vi "MGCC_StaEst_complex2magnitude.vi"(10 "st_MGCC_StaEst_Input":T1) -> (2 "output cluster":T1)   [LabVIEW 2016]
doc: "-----------------------------------------------------------------------------------------------------------------------\nCopyright <2019> <The University of Tennessee at Knoxville and the University of Tennessee Research Foundation>\nThis software is released under BSD-3 \nhttps://opensource.org/licenses/BSD-3-Clause \nAdditional license options available at https://utrf.tennessee.edu/industry/sample-agreements/\n-----------------------------------------------------------------------------------------------------------------------"
uses:
  Model Management/Global_MdlMgmt.vi
  Communication/Global communication.vi
  <vilib>/imath/engines/lvmath2/RunTimeEngine/IndexRead/NIMS M($,S).vi
  <instcachedir>/0/NIMS M($,S)_3E5749BBB62E49528D4765A77F1F6D98.lvgen/NIMS M($,S)_3E5749BBB62E49528D4765A77F1F6D98_000.vi
  <vilib>/imath/engines/lvmath2/RunTimeEngine/BuiltInFunctions/length/NIMS_length(GV).vi
  <instcachedir>/0/NIMS_length(GV)_08A3D13377FD4E4B96F5795FBF3698FA.lvgen/NIMS_length(GV)_08A3D13377FD4E4B96F5795FBF3698FA_000.vi
  <vilib>/imathl/engines/lvmath/Functions/Error Handling/Create Error.vi
  <vilib>/imath/engines/lvmath2/RunTimeEngine/RangeToken/NIMS_Range_R3 - Integer.vi
  <instcachedir>/0/NIMS_Range_R3 - Integer_A435E2FF893B4C718FD5055FE39FE2F6.lvgen/NIMS_Range_R3 - Integer_A435E2FF893B4C718FD5055FE39FE2F6_000.vi
  <vilib>/imath/engines/lvmath2/RunTimeEngine/CommandStatement/MC_CommandStatement_break.vi
  <vilib>/imath/engines/lvmath2/RunTimeEngine/IndexRead/NIMS M(S,S).vi
  <instcachedir>/0/NIMS M(S,S)_AC51E74150A542F7991B9634C66F3096.lvgen/NIMS M(S,S)_AC51E74150A542F7991B9634C66F3096_000.vi
  <vilib>/imath/engines/lvmath2/RunTimeSupport/NIMS_Error if Not Equal.vi
  <instcachedir>/0/NIMS_Error if Not Equal_43252A79AD05436189442EC0C5E5AB8A.lvgen/NIMS_Error if Not Equal_43252A79AD05436189442EC0C5E5AB8A_000.vi
  <vilib>/imath/engines/lvmath2/RunTimeEngine/IndexRead/NIMS V(S).vi
  <instcachedir>/0/NIMS V(S)_0488751826AF41519A22953C041130DC.lvgen/NIMS V(S)_0488751826AF41519A22953C041130DC_000.vi
  <vilib>/imath/engines/lvmath2/RunTimeEngine/IndexReplace/NIMS M(S,S)=S.vi
  <instcachedir>/0/NIMS M(S,S)=S_98E40400474E4398B113AE20298B4F82.lvgen/NIMS M(S,S)=S_98E40400474E4398B113AE20298B4F82_000.vi
  <vilib>/imath/engines/lvmath2/RunTimeEngine/ErrorHandling/NIMS_Create Error From Enums.vi
  <vilib>/imath/engines/lvmath2/RunTimeEngine/NodeEndStatement/NIMS_NodeEndStatement_Output.vi
  <instcachedir>/0/NIMS_NodeEndStatement_Output_53EC0D466D134D7ABD903AC30B43404B.lvgen/NIMS_NodeEndStatement_Output_53EC0D466D134D7ABD903AC30B43404B_002.vi
  <vilib>/imath/engines/lvmath2/RunTimeEngine/ErrorHandling/NIMS_Finalize Error.vi
  <vilib>/Utility/error.llb/Error Cluster From Error Code.vi
  <vilib>/ErrorRing/Error Ring.xnode
panel:
  out "error out":errorcluster
  out "appended array":dbl[][](array[numeric])
  out "V_node":cdb[][](array[numeric])
  out "r * e^(i*theta)":cdb[][](array[numeric])
  out "output array":dbl[][](array[numeric])
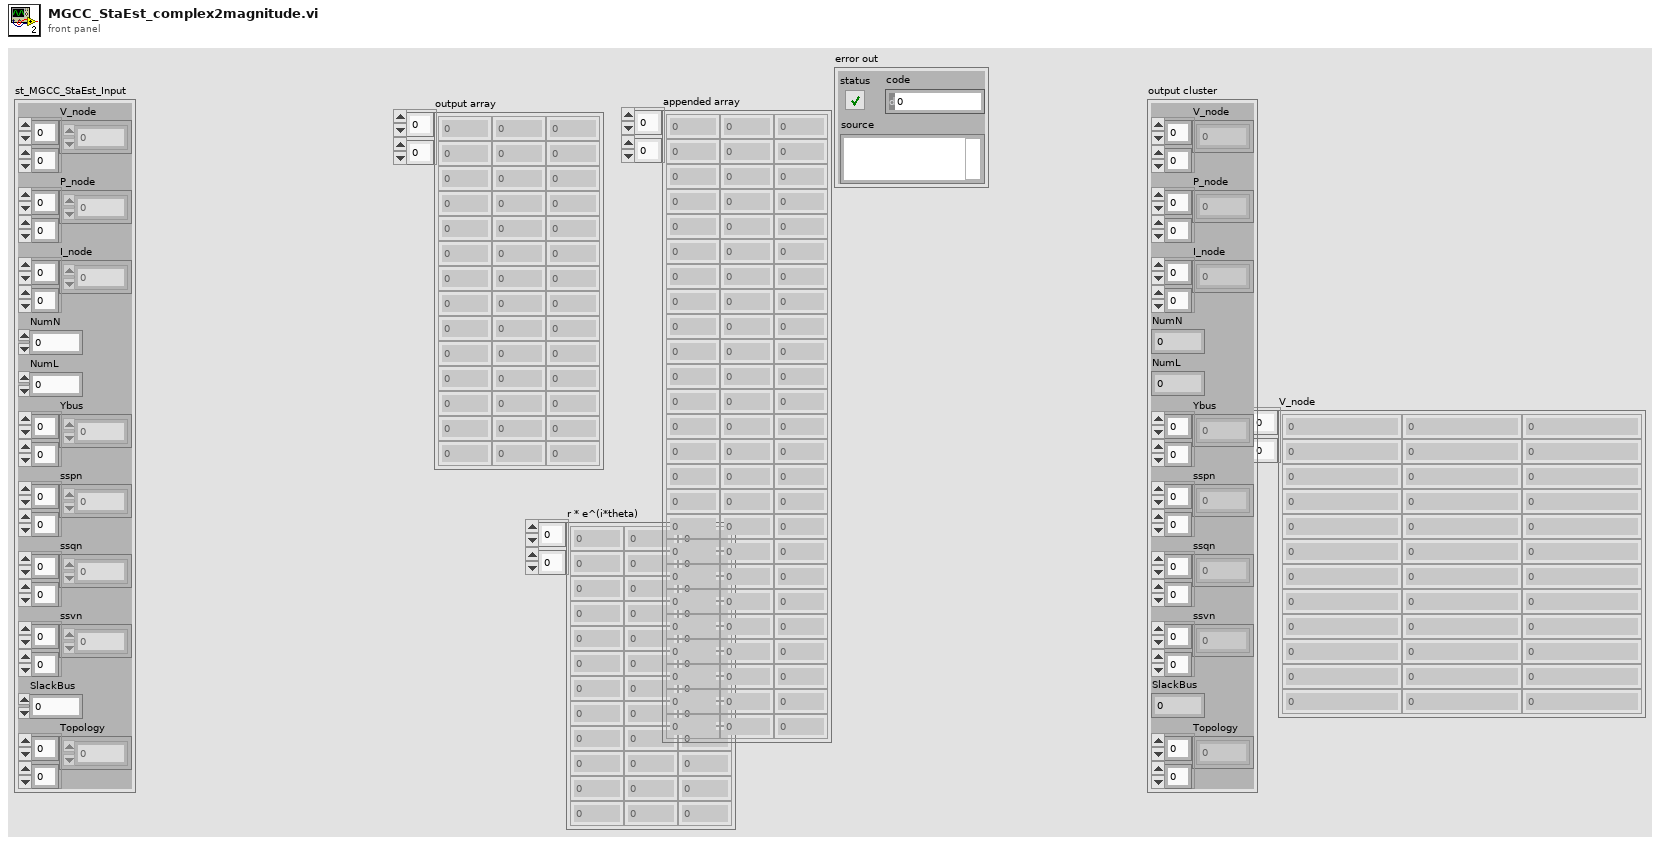
[diagram p1: front panel]
types:
  T1 = cluster{"V_node":cdb[][], "P_node":cdb[][], "I_node":cdb[][], "NumN":dbl, "NumL":dbl, "Ybus":cdb[][], "sspn":dbl[][], "ssqn":dbl[][], "ssvn":dbl[][], "SlackBus":dbl, "Topology":dbl[][]}
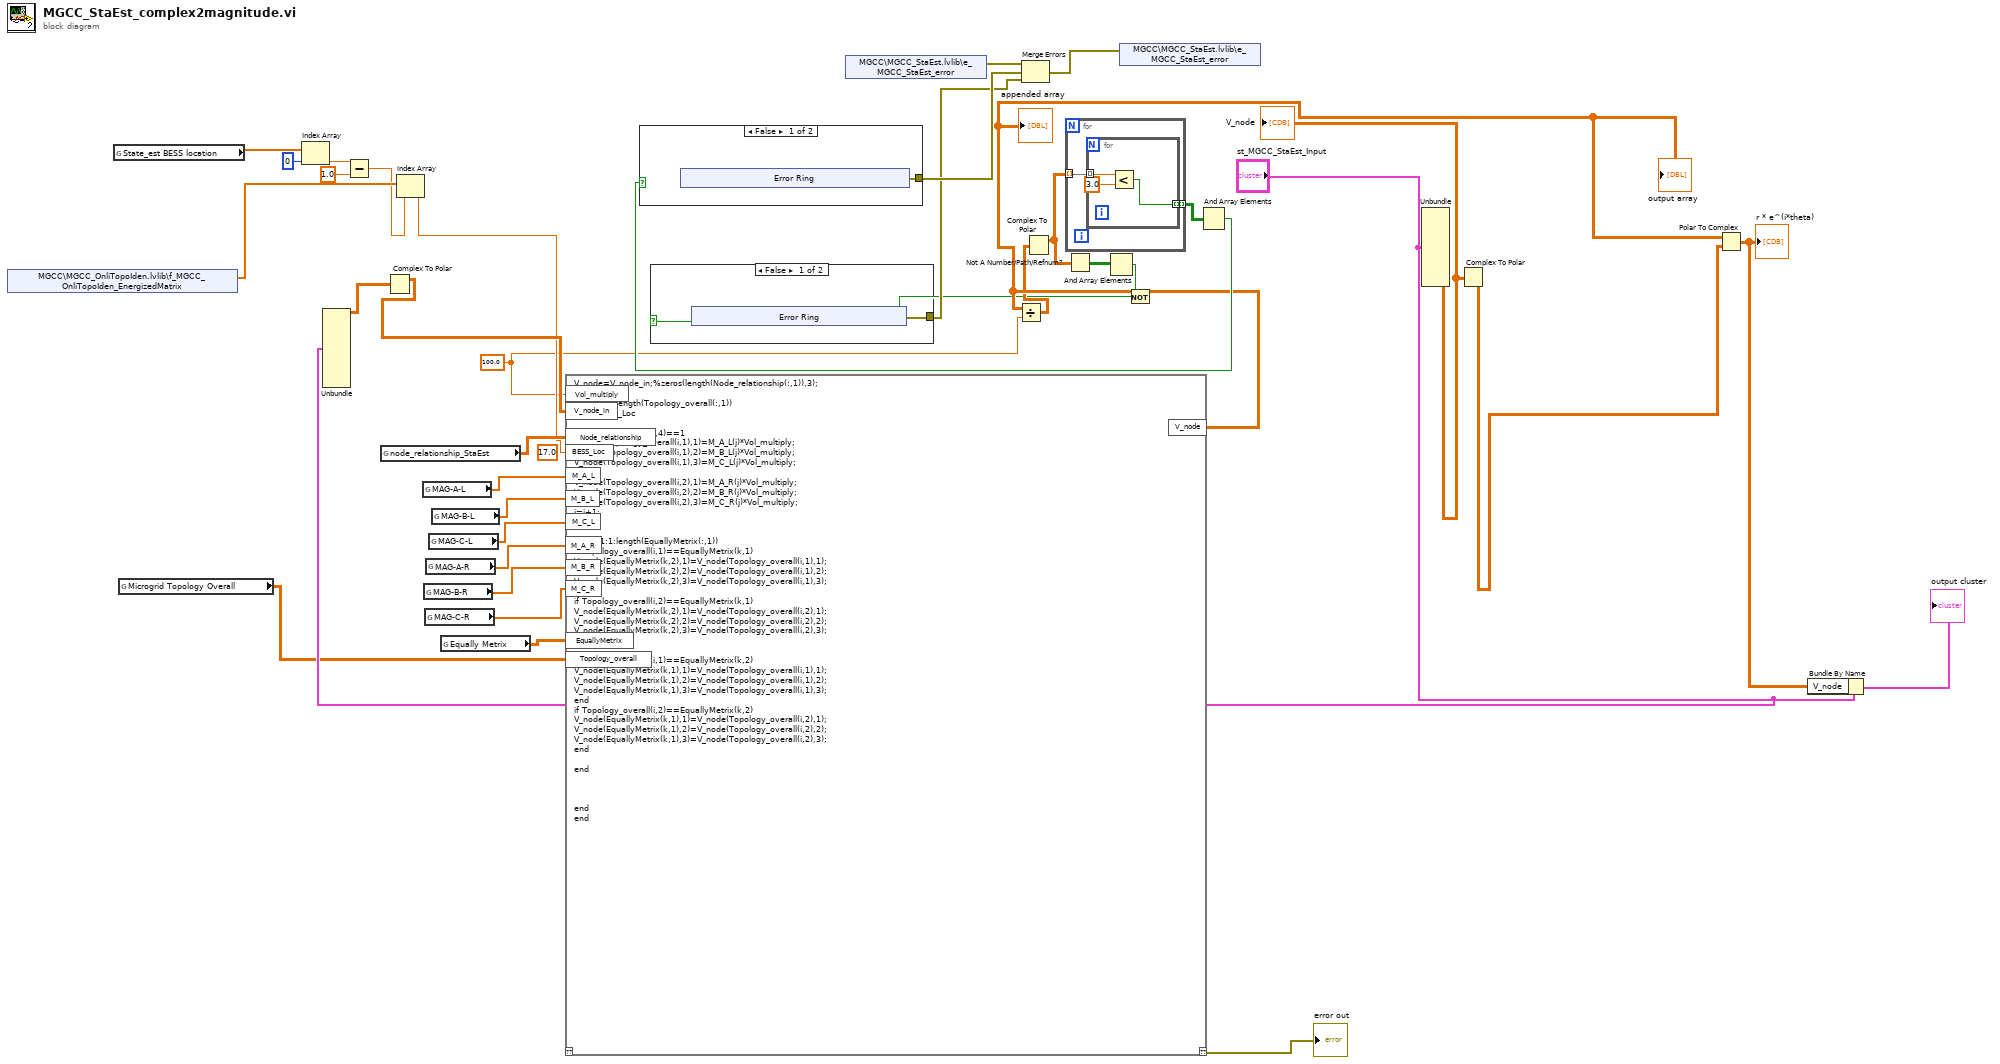
[diagram p0: block diagram]
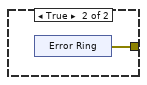
[diagram p2: hidden frame]
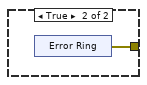
[diagram p3: hidden frame]
diagram:
  (unwired) 17.0 ("BESS_Loc")
  w3 = 100.0 ("y")
  n1 = shared-variable "MGCC\\MGCC_OnliTopoIden.lvlib\\f_MGCC_OnliTopoIden_EnergizedMatrix"() -> (w21:dbl[])  [unwired: 1 in, 1 out]
  n2 = global read "Global_MdlMgmt.vi" "State_est BESS location"() -> (w23:dbl[])
  n3 = global read "Global_MdlMgmt.vi" "Microgrid Topology Overall"() -> (w19:dbl[][])
  n4 = Index Array(array=w23, index=0) -> (element=w17:dbl)
  n5 = Unbundle("st_MGCC_StaEst_Input") -> ("V_node"=w33:cdb[][])  [unwired: 10 out]
  n6 = Subtract(x=w17, y=1.0) -> (x-y=w15:dbl)
  n7 = global read "Global_MdlMgmt.vi" "node_relationship_StaEst"() -> (w32:dbl[][])
  n8 = Complex To Polar(r * e^(i*theta)=w33) -> (r=w25:dbl[][])  [unwired: 1 out]
  n9 = Index Array(array=w21, index=w15) -> (element=w18:dbl)
  n10 = global read "Global communication.vi" "MAG-A-L"() -> (w31:dbl[])
  n11 = global read "Global communication.vi" "MAG-B-R"() -> (w27:dbl[])
  n12 = global read "Global communication.vi" "MAG-C-R"() -> (w26:dbl[])
  n13 = global read "Global communication.vi" "MAG-A-R"() -> (w28:dbl[])
  n14 = global read "Global communication.vi" "MAG-C-L"() -> (w29:dbl[])
  n15 = global read "Global communication.vi" "MAG-B-L"() -> (w30:dbl[])
  n16 = global read "Global_MdlMgmt.vi" "Equally Metrix"() -> (w20:dbl[][])
  n17 = mathscript code="V_node=V_node_in;%zeros(length(Node_relationship(:,1)),3);\nj=1;\nfor i =1:1:length(Topology_overall(:,1))\nif i~=BESS_Loc\n\nif Topology_overall(i,4)==1\nV_node(Topology_overall(i,1),1)=M_A_L(j)*Vol_multiply;\nV_node(Topology_overall(i,1),2)=M_B_L(j)*Vol_multiply;\nV_node(Topology_overall(i,1),3)=M_C_L(j)*Vol_multiply;\n\nV_node(Topology_overall(i,2),1)=M_A_R(j)*Vol_multiply;\nV_node(Topology_overall(i,2),2)=M_B_R(j)*Vol_multiply;\nV_node(Topology_overall(i,2),3)=M_C_R(j)*Vol_multiply;\nj=j+1;\nend\n\nfor k=1:1:length(EquallyMetrix(:,1))\nif Topology_overall(i,1)==EquallyMetrix(k,1)\nV_node(EquallyMetrix(k,2),1)=V_node(Topology_overall(i,1),1);\nV_node(EquallyMetrix(k,2),2)=V_node(Topology_overall(i,1),2);\nV_node(EquallyMetrix(k,2),3)=V_node(Topology_overall(i,1),3);\nend\nif Topology_overall(i,2)==EquallyMetrix(k,1)\nV_node(EquallyMetrix(k,2),1)=V_node(Topology_overall(i,2),1);\nV_node(EquallyMetrix(k,2),2)=V_node(Topology_overall(i,2),2);\nV_node(EquallyMetrix(k,2),3)=V_node(Topology_overall(i,2),3);\nend\n\nif Topology_overall(i,1)==EquallyMetrix(k,2)\nV_node(EquallyMetrix(k,1),1)=V_node(Topology_overall(i,1),1);\nV_node(EquallyMetrix(k,1),2)=V_node(Topology_overall(i,1),2);\nV_node(EquallyMetrix(k,1),3)=V_node(Topology_overall(i,1),3);\nend\nif Topology_overall(i,2)==EquallyMetrix(k,2)\nV_node(EquallyMetrix(k,1),1)=V_node(Topology_overall(i,2),1);\nV_node(EquallyMetrix(k,1),2)=V_node(Topology_overall(i,2),2);\nV_node(EquallyMetrix(k,1),3)=V_node(Topology_overall(i,2),3);\nend\n\nend\n\n\n\nend\nend"("Node_relationship"=w32, "Vol_multiply"=w3, "M_A_L"=w31, "M_B_L"=w30, "M_C_L"=w29, "M_A_R"=w28, "M_B_R"=w27, "M_C_R"=w26, "V_node_in"=w25, "BESS_Loc"=w18, "EquallyMetrix"=w20, "Topology_overall"=w19) -> ("??"=→"error out":errorcluster, "V_node"=w4:dbl[][])  [unwired: 1 in]
  "output array" <- w4
  "appended array" <- w4
  n18 = shared-variable "MGCC\\MGCC_StaEst.lvlib\\e_MGCC_StaEst_error"() -> (w14:errorcluster)  [unwired: 1 in, 1 out]
  n19 = Divide(x=w4, y=w3) -> (x/y=w2:dbl[][])
  n20 = Complex To Polar(r * e^(i*theta)=w2) -> (r=w8:dbl[][])  [unwired: 1 out]
  n21 = for {
    tunnel: w8 -> [w39] mode=indexing
    tunnel: [w38] -> w7 mode=indexing
    n22 = for {
      tunnel: w39 -> [w42] mode=indexing
      tunnel: [w40] -> w38 mode=indexing
      n23 = Less?(x=w42, y=3.0) -> (x < y?=w40:bool)
    }
  }
  n24 = Not A Number/Path/Refnum?(number/path/refnum=w8) -> (NaN/Path/Refnum?=w11:bool[][])
  n25 = And Array Elements(Boolean array=w11) -> (logical AND=w10:bool)
  n26 = Not(x=w10) -> (.not. x?=w1:bool)
  n27 = case shown="False" w1 {
    tunnel: [w43 w49] -> w9
    frame False {
      n28 = xnode "Error Ring"() -> ("error out"=w43:errorcluster)
    }
    frame True {
      n29 = xnode "Error Ring"() -> ("error out"=w49:errorcluster)
    }
  }
  n30 = And Array Elements(Boolean array=w7) -> (logical AND=w6:bool)
  n31 = case shown="False" w6 {
    tunnel: [w51 w57] -> w12
    frame False {
      n32 = xnode "Error Ring"() -> ("error out"=w51:errorcluster)
    }
    frame True {
      n33 = xnode "Error Ring"() -> ("error out"=w57:errorcluster)
    }
  }
  n34 = Merge Errors(w14, w12, w9) -> (w13:errorcluster)
  n35 = shared-variable "MGCC\\MGCC_StaEst.lvlib\\e_MGCC_StaEst_error"(w13) -> ()  [unwired: 1 in, 1 out]
  n36 = Unbundle("st_MGCC_StaEst_Input") -> ("V_node"=w35:cdb[][])  [unwired: 10 out]
  "V_node" <- w35
  n37 = Complex To Polar(r * e^(i*theta)=w35) -> (theta=w34:dbl[][])  [unwired: 1 out]
  n38 = Polar To Complex(1:w34, 2:w4) -> (0:w37:cdb[][])
  "r * e^(i*theta)" <- w37
  n39 = Bundle By Name(cluster="st_MGCC_StaEst_Input", "V_node"=w37) -> (→"output cluster":T1)
